vi "connect.vi"(7 "server name":string, 8 "error in":errorcluster, 10 "connection ID":refnum<k5>, 11 "lvlibretls client socket":refnum<class "lvlibretls client socket.lvclass">) -> (0 "error out":errorcluster, 2 "lvlibretls connection":refnum<class "lvlibretls connection.lvclass">, 3 "lvlibretls client socket out":refnum<class "lvlibretls client socket.lvclass">)   [LabVIEW 2016, in "lvlibretls client socket.lvclass"]
doc: "Creates a socket context in the client configuration using an initialized labview tcp socket. The server name field is used for verification."
uses:
  lvlibretls client socket.lvclass
  C:/Users/IEUser/Desktop/tlssimple/libretls/context parent/lvlibretls configurable context.lvclass
  socket connection/lvlibretls connection.lvclass
  context parent/lvlibretls configurable context.lvclass/lvlibretls configurable context.ctl
  lv tls dll.lvlib
  context parent/lvlibretls configurable context.lvclass
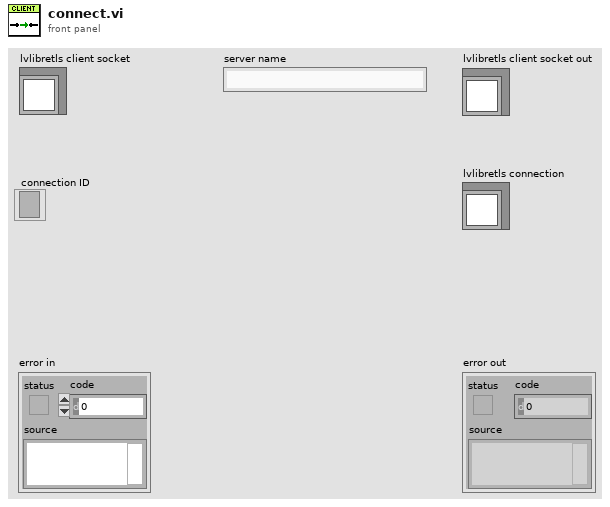
[diagram p1: front panel]
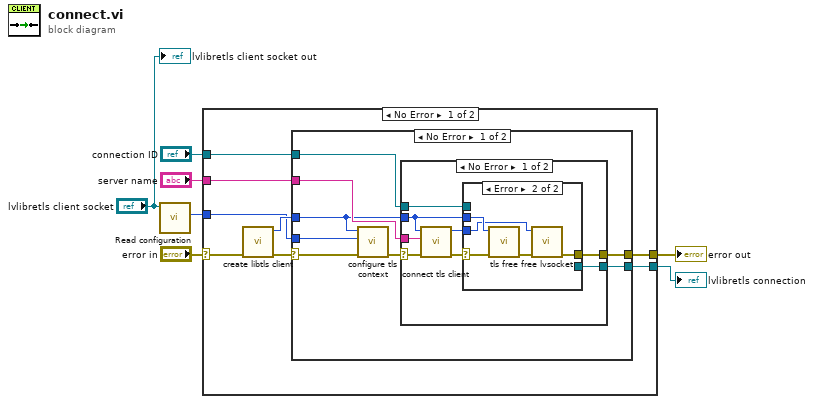
[diagram p0: block diagram]
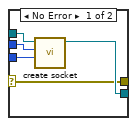
[diagram p2: hidden frame]
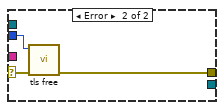
[diagram p3: hidden frame]
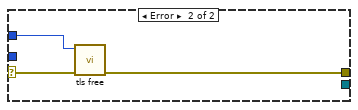
[diagram p4: hidden frame]
diagram:
  n1 = call "Read configuration.vi"("lvlibretls configurable context in"="lvlibretls client socket") -> ("configuration"=w1:u64)  [unwired: 10 in]
  n2 = case shown="No Error" "error in" {
    selector: "error in" -> [w10 w48]
    tunnel: [w15 w48] -> w7
    tunnel: "server name" -> [w14 _]
    tunnel: "connection ID" -> [w13 _]
    tunnel: [w12 _] -> w4
    tunnel: w1 -> [w8 _]
    frame No Error {
      n3 = call "create libtls client.vi"("error in"=w10) -> ("error out"=w11:errorcluster, "client out"=w9:u64)  [unwired: 9 in]
      n4 = case shown="No Error" w11 {
        selector: w11 -> [w19 w47]
        tunnel: [w23 w46] -> w15
        tunnel: w14 -> [w22 _]
        tunnel: w13 -> [w21 _]
        tunnel: [w20 _] -> w12
        tunnel: w9 -> [w17 w45]
        tunnel: w8 -> [w16 _]
        frame No Error {
          n5 = call "configure tls context.vi"("error in"=w19, "config"=w16, "context"=w17) -> ("error out"=w18:errorcluster)  [unwired: 8 in]
          n6 = case shown="No Error" w18 {
            selector: w18 -> [w27 w44]
            tunnel: [w24 w43] -> w23
            tunnel: w22 -> [w31 _]
            tunnel: w21 -> [w30 _]
            tunnel: [w28 _] -> w20
            tunnel: w17 -> [w26 w42]
            frame No Error {
              n7 = call "connect tls client.vi"("error in"=w27, "servername"=w31, "client"=w26) -> ("error out"=w25:errorcluster, "lvsocket"=w29:u64)  [unwired: 7 in]
              n8 = case shown="Error" w25 {
                selector: w25 -> [w32 w41]
                tunnel: w30 -> [w36 _]
                tunnel: w29 -> [w35 w37]
                tunnel: [w34 _] -> w28
                tunnel: w26 -> [w33 w38]
                tunnel: [w32 w39] -> w24
                frame No Error {
                  n9 = call "create socket.vi"("lvsocket"=w35, "tls socket"=w33, "connection"=w36) -> ("lvlibretls connection out"=w34:refnum<class "lvlibretls connection.lvclass">)  [unwired: 8 in]
                }
                frame Error {
                  n10 = call "tls free.vi"("error in"=w41, "tls context"=w38) -> ("error out"=w40:errorcluster)  [unwired: 9 in]
                  n11 = call "free lvsocket.vi"("error in"=w40, "lvsocket"=w37) -> ("error out"=w39:errorcluster)  [unwired: 9 in]
                }
              }
            }
            frame Error {
              n12 = call "tls free.vi"("error in"=w44, "tls context"=w42) -> ("error out"=w43:errorcluster)  [unwired: 9 in]
            }
          }
        }
        frame Error {
          n13 = call "tls free.vi"("error in"=w47, "tls context"=w45) -> ("error out"=w46:errorcluster)  [unwired: 9 in]
        }
      }
    }
    frame Error {
    }
  }
  "error out" <- w7
  "lvlibretls connection" <- w4
  "lvlibretls client socket out" <- "lvlibretls client socket"
